vi "Lithographify_funnel&rec.vi"(5 "Data In":cluster{string, cluster{"X":dbl, "Y":dbl}[]}, 7 "Direction":u16, 9 "Speed (µm/s)":T2={"Schedule"=enum."Constant", "Settings"=variant(dbl 0.0)}, 11 "Voltage (V)":T2={"Schedule"=enum."Constant", "Settings"=variant(dbl 0.0)}, 12 "Set Resistance":T1=enum."1G ohm", 13 "Enabled":bool) -> (4 "Lithography Data":T4={"Name"="", "Litho"=[], "Set Resistance"=enum."1G ohm"})   [LabVIEW 2019]
doc: "This VI calculates the lithography data of one pattern and organizes it appropriately."
uses:
  <userlib>/LevyLab/Relay Box/Typedefs/Resistor--enum.ctl
  typedefs/Voltage - cluster.ctl
  typedefs/Schedule - enum.ctl
  <userlib>/LevyLab/Relay Box/Relay-Box.lvclass
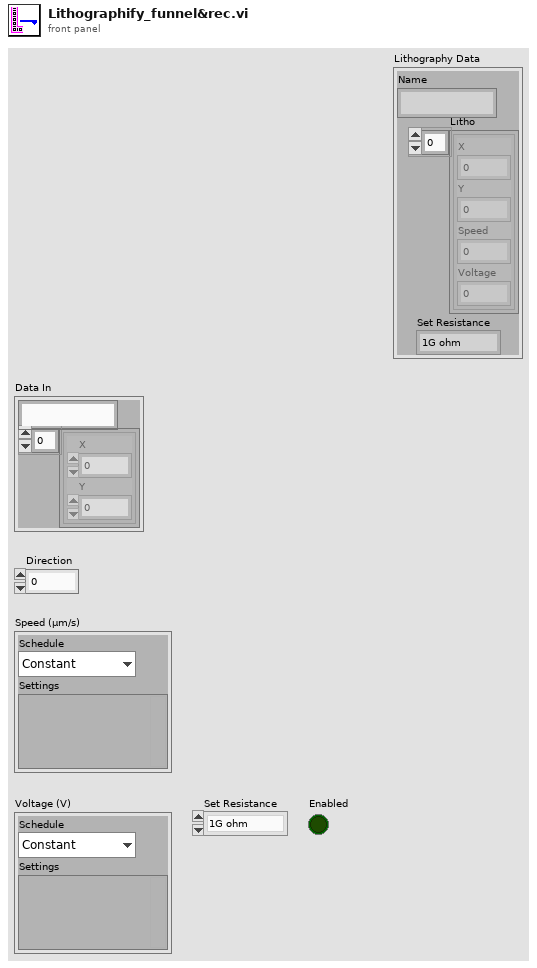
[diagram p1: front panel]
types:
  T1 = typedef "Relay-Box.lvclass/Resistor--enum.ctl" = enum16{"open", "discharge tip", "0 ohms", "100k ohm", "10M ohm", "1G ohm"}
  T2 = typedef "Voltage - cluster.ctl" = cluster{"Schedule":T3, "Settings":variant}
  T3 = typedef "Schedule - enum.ctl" = enum16{"Constant", "Ramp", "Fn. Generator", "Formula"}
  T4 = cluster{"Name":string, "Litho":cluster{"X":dbl, "Y":dbl, "Speed":dbl, "Voltage":dbl}[], "Set Resistance":T1}
  T5 = cluster{"X":dbl, "Y":dbl, "Speed":dbl, "Voltage":dbl}[]
  T6 = cluster{"X":dbl, "Y":dbl, "Speed":dbl, "Voltage":dbl}
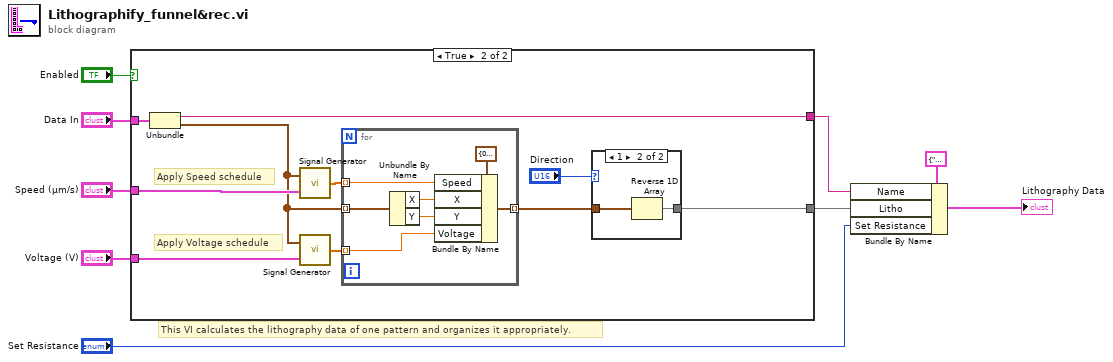
[diagram p0: block diagram]
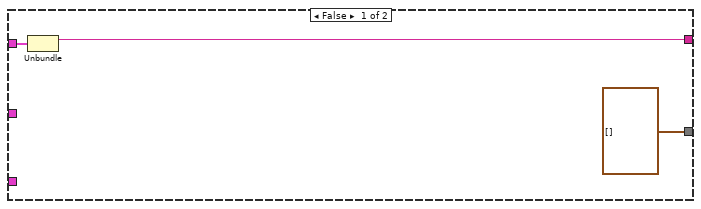
[diagram p2: hidden frame]
diagram:
  # "This VI calculates the lithography data of one pattern and organizes it appropriately."
  n1 = case shown="True" "Enabled" {
    tunnel: [w11 w13] -> w9
    tunnel: "Data In" -> [w12 w22]
    tunnel: "Voltage (V)" -> [_ w19]
    tunnel: "Speed (µm/s)" -> [_ w18]
    tunnel: [T5 [] w16] -> w3
    frame False {
      n2 = Unbundle(w12) -> (w11:string)  [unwired: 1 out]
    }
    frame True {
      # "Apply Voltage schedule"
      # "Apply Speed schedule"
      n3 = Unbundle(w22) -> (w13:string, w14:cluster{"X":dbl, "Y":dbl}[])
      n4 = call "Signal Generator.vi"("Signal Properties"=w18, "Points"=w14) -> ("Signal"=w20:dbl[])
      n5 = call "Signal Generator.vi"("Signal Properties"=w19, "Points"=w14) -> ("Signal"=w21:dbl[])
      n6 = for {
        tunnel: w20 -> [w26] mode=indexing
        tunnel: w21 -> [w29] mode=indexing
        tunnel: w14 -> [w31] mode=indexing
        tunnel: [w28] -> w17 mode=indexing
        n7 = Unbundle By Name(w31) -> ("X"=w32:dbl, "Y"=w30:dbl)
        n8 = Bundle By Name(cluster=T6 {"X"=0.0, "Y"=0.0, "Speed"=0.0, "Voltage"=0.0} ("Litho Point"), "Speed"=w26, "X"=w32, "Y"=w30, "Voltage"=w29) -> (w28:T6)
      }
      n9 = case shown="1" "Direction" {
        tunnel: w17 -> [w23 w25]
        tunnel: [w23 w24] -> w16
        frame 0, Default {
        }
        frame 1 {
          n10 = Reverse 1D Array(array=w25) -> (reversed array=w24:T5)
        }
      }
    }
  }
  n11 = Bundle By Name(cluster=T4 {"Name"="", "Litho"=[], "Set Resistance"=enum."1G ohm"} ("Lithography Data"), "Name"=w9, "Litho"=w3, "Set Resistance"="Set Resistance") -> (→"Lithography Data":T4)
